vi "Reinit_to_Default_on_Multiple_Controls.vi"(11 "配列":refnum<vi>[](array[refnum])) -> ()   [LabVIEW 2017]
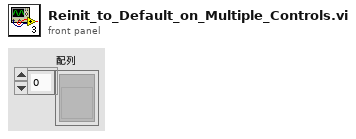
[diagram p1: front panel]
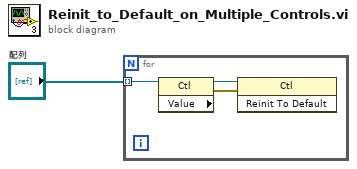
[diagram p0: block diagram]
diagram:
  n1 = for {
    tunnel: "配列" -> [w4] mode=indexing
    n2 = property class="Ctl" props=["Value"](reference=w4) -> (reference out=w3:refnum<vi>, error out=w2:errorcluster)  [unwired: 1 in, 1 out]
    n3 = invoke class="Ctl" method="Reinit To Default"(reference=w3, error in=w2) -> ()  [unwired: 1 in, 3 out]
  }
